vi "DataType2.vi"(11 "DataName":string) -> (1 "isBool?":bool, 2 "datatype":string, 3 "DataName(dup)":string)   [LabVIEW 2020, in "CSM-TagDashboard.lvlib"]
uses:
  CSM-TagDashboard.lvlib
  <userlib>/_NEVSTOP/Communicable State Machine(CSM)/addons/INI-Static-Variable-Support/INI-Static-Variable-Support.lvlib
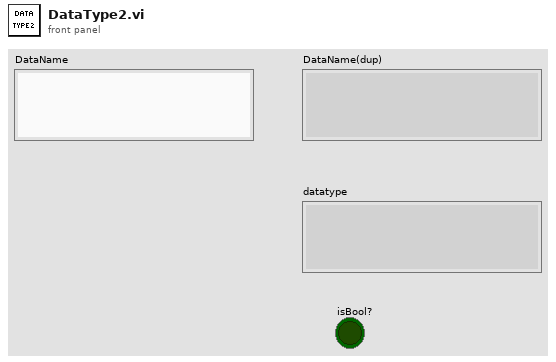
[diagram p1: front panel]
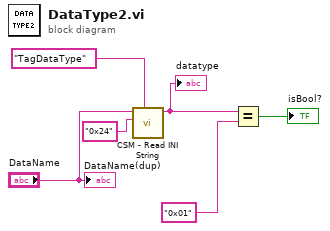
[diagram p0: block diagram]
diagram:
  n1 = call <userlib>:"CSM - Read INI String.vi"("Section Name (\"\" as Default)"="TagDataType" ("Section Name(\"\" as Default)"), "Default Value"="0x24" ("y"), "Variable Name"="DataName") -> ("Value"=w5:string)  [unwired: 4 in, 2 out]
  "datatype" <- w5
  n2 = Equal?(x=w5, y="0x01") -> (x = y?=→"isBool?":bool)
  "DataName(dup)" <- "DataName"
